vi "Forward Lockin Result to Output.vi"(8 "error in (no error)":errorcluster, 10 "Waveforms [] in":waveform(dbl)[](array[waveform]), 11 "Instrument.DAQ in":refnum<class "Instrument.DAQ.lvclass">) -> (0 "error out":errorcluster, 2 "Waveforms [] out":waveform(dbl)[](array[waveform]), 3 "Instrument.DAQ out":refnum<class "Instrument.DAQ.lvclass">)   [LabVIEW 2019, in "Instrument.DAQ.lvclass"]
uses:
  Instrument.DAQ.lvclass
  Instrument.Lockin/Typedefs/Results Type--Enum.ctl
  Instrument.Lockin/Instrument.Lockin.lvclass
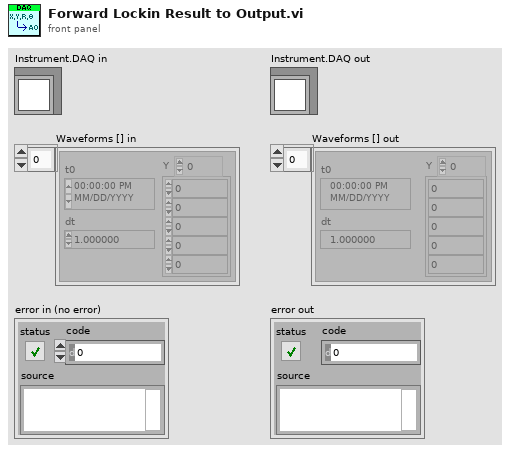
[diagram p1: front panel]
types:
  T1 = typedef "Instrument.Lockin.lvclass/Results Type--Enum.ctl" = enum16{"X", "Y", "R", "Theta", "Mean"}
  T2 = typedef "Instrument.DAQ.lvclass/DAQ.Config.AO--Cluster--Array.ctl" = T3[]
  T3 = typedef "Instrument.DAQ.lvclass/DAQ.Config.AO--Cluster.ctl" = cluster{"Channels":tag, "Range":T4, "output terminal configuration":i32, "Type":T5}
  T4 = typedef "Instrument.DAQ.lvclass/DAQ.Config.AO.Range--enum.ctl" = enum16{"±0.1", "±1.0", "±10.0"}
  T5 = typedef "Instrument.DAQ.lvclass/DAQ.Type--enum.ctl" = enum16{"None", "USB-4431", "PXI-446x"}
  T6 = typedef "Instrument.DAQ.lvclass/DAQ.Config.AI--Cluster--Array.ctl" = T7[]
  T7 = typedef "Instrument.DAQ.lvclass/DAQ.Config.AI--Cluster.ctl" = cluster{"Channels":tag, "Coupling":T8, "Range":T9, "input terminal configuration":i32, "Type":T5}
  T8 = typedef "Instrument.DAQ.lvclass/DAQ.Config.AI.Coupling--enum.ctl" = u16
  T9 = typedef "Instrument.DAQ.lvclass/DAQ.Config.AI.Range--enum.ctl" = enum16{"±0.316", "±1.00", "±3.16", "±10.0", "±31.6", "±42.4"}
  T10 = typedef "Instrument.DAQ.lvclass/AI.Channel--Cluster--Array.ctl" = T11[]
  T11 = typedef "Instrument.DAQ.lvclass/AI.Channel--Cluster.ctl" = cluster{"Enable?":bool, "Channel":i32, "References":i32[]}
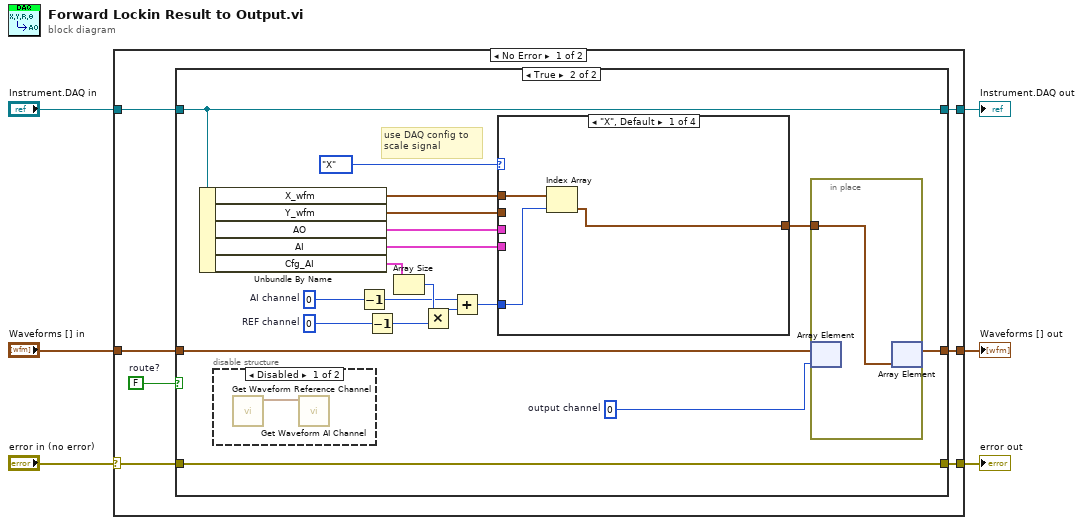
[diagram p0: block diagram]
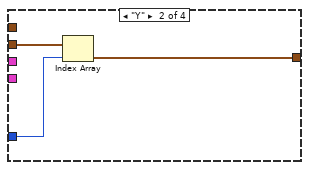
[diagram p3: hidden frame]
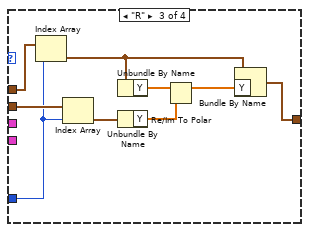
[diagram p4: hidden frame]
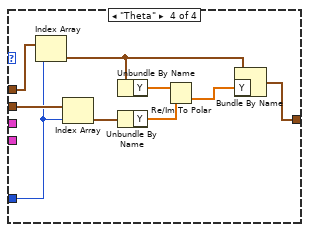
[diagram p5: hidden frame]
diagram:
  n1 = case shown="No Error" "error in (no error)" {
    selector: "error in (no error)" -> [w11 w64]
    tunnel: [w12 w64] -> w1
    tunnel: [w9 w63] -> w3
    tunnel: "Instrument.DAQ in" -> [w13 w63]
    tunnel: "Waveforms [] in" -> [w7 w62]
    tunnel: [w8 w62] -> w6
    frame No Error {
      w10 = FALSE  # route?
      n2 = case shown="True" w10 {
        tunnel: w13 -> [w16 w34]
        tunnel: [w14 w35] -> w12
        tunnel: w11 -> [w14 w35]
        tunnel: [w16 w34] -> w9
        tunnel: [w15 w22] -> w8
        tunnel: w7 -> [w15 w24]
        frame False {
        }
        frame True {
          w23 = 0  # output channel
          w27 = 0  # REF channel
          w31 = 0  # AI channel
          # "use DAQ config to\nscale signal"
          n3 = Unbundle By Name(w34) -> ("X_wfm"=w32:waveform(dbl)[], "Y_wfm"=w19:waveform(dbl)[], "AO"=w18:T2, "AI"=w17:T6, "Cfg_AI"=w30:T10)
          n4 = disable-structure shown="Disabled" {
            frame Disabled {
              n5 = call "Get Waveform Reference Channel.vi"() -> ("Reference out"=w61:waveform(dbl))  [unwired: 9 in, 2 out]
              n6 = call "Get Waveform AI Channel.vi"("Reference in"=w61) -> ()  [unwired: 8 in, 3 out]
            }
            frame Enabled {
            }
          }
          n7 = Decrement(x=w31) -> (x-1=w25:i32)
          n8 = Decrement(x=w27) -> (x-1=w26:i32)
          n9 = Array Size(array=w30) -> (size(s)=w28:i32)
          n10 = Multiply(x=w28, y=w26) -> (x*y=w29:i32)
          n11 = Add(x=w25, y=w29) -> (x+y=w20:i32)
          n12 = case shown="\"X\", Default" Results_Type--Enum."X" ("Type") {
            tunnel: [w37 w41 w44 w54] -> w33
            tunnel: w32 -> [w38 _ w49 w58]
            tunnel: w20 -> [w36 w39 w48 w57]
            tunnel: w19 -> [_ w40 w50 w59]
            tunnel: w18 -> [_ _ _ _]
            tunnel: w17 -> [_ _ _ _]
            frame "X", Default {
              n13 = Index Array(array=w38, index=w36) -> (element=w37:waveform(dbl))
            }
            frame "Y" {
              n14 = Index Array(array=w40, index=w39) -> (element=w41:waveform(dbl))
            }
            frame "R" {
              n15 = Index Array(array=w49, index=w48) -> (element=w42:waveform(dbl))
              n16 = Index Array(array=w50, index=w48) -> (element=w43:waveform(dbl))
              n17 = Unbundle By Name(w42) -> ("Y"=w47:dbl[])
              n18 = Unbundle By Name(w43) -> ("Y"=w46:dbl[])
              n19 = Re/Im To Polar(2:w46, 3:w47) -> (1:w45:dbl[])  [unwired: 1 out]
              n20 = Bundle By Name(cluster=w42, "Y"=w45) -> (w44:waveform(dbl))
            }
            frame "Theta" {
              n21 = Index Array(array=w58, index=w57) -> (element=w52:waveform(dbl))
              n22 = Index Array(array=w59, index=w57) -> (element=w53:waveform(dbl))
              n23 = Unbundle By Name(w52) -> ("Y"=w56:dbl[])
              n24 = Unbundle By Name(w53) -> ("Y"=w55:dbl[])
              n25 = Re/Im To Polar(2:w55, 3:w56) -> (0:w51:dbl[])  [unwired: 1 out]
              n26 = Bundle By Name(cluster=w52, "Y"=w51) -> (w54:waveform(dbl))
            }
          }
          n27 = in-place {
            in-place-border: w33 -> [w60]
            n28 = in-place-array #1(w24, w23) -> ()  [unwired: 1 out]
            n29 = in-place-array #1(w60) -> (w22:waveform(dbl)[])  [unwired: 1 out]
          }
        }
      }
    }
    frame Error {
    }
  }
  "Waveforms [] out" <- w6
  "Instrument.DAQ out" <- w3
  "error out" <- w1
